vi "sub_Filter_Waveforms_by_Channel_and_Time.vi"(6 "End Time":timestamp, 7 "Start Time":timestamp, 8 "error in":errorcluster, 9 "Channel Key":string, 10 "Waveforms in":T3[](array[typedef]), 11 "daq.io type in":T1={"daq.io ref"=refnum, "daq.io API Base"="http://dashboard.daq.io/api/v1", "Device Key"="", "Account ID"="", "online"=TRUE, "SSL"=TRUE}) -> (0 "error out":errorcluster, 2 "Filtered Waveforms out":T3[](array[typedef]), 3 "daq.io type out":T1={"daq.io ref"=refnum, "daq.io API Base"="http://dashboard.daq.io/api/v1", "Device Key"="", "Account ID"="", "online"=TRUE, "SSL"=TRUE})   [LabVIEW 2013, in "daqio minimal.lvlib"]
doc: "This VI filters existing waveforms by date and channel name and returns only the ones specified by the user. If no start time is specified, all entries before end time will be returned. If no end time is specified, all entries after start time are specified. If neither start nor end time are specified, all entries will be returned. Pass \"*\" as Channel Key if you would like to return all Channels"
uses:
  daqio minimal.lvlib
  _typedefs/daqio-read-waveform-JSON-header-time.ctl
  _typedefs/daqio-Type.ctl
  <vilib>/httpClient/ClientHandle.ctl
  _typedefs/daqio-Device.ctl
  _typedefs/daqio-Channels.ctl
  _typedefs/daqio-Device-Dashboards.ctl
  <vilib>/Easy HTTP Client/Easy HTTP.lvlib
  <vilib>/httpClient/LabVIEWHTTPClient.lvlib
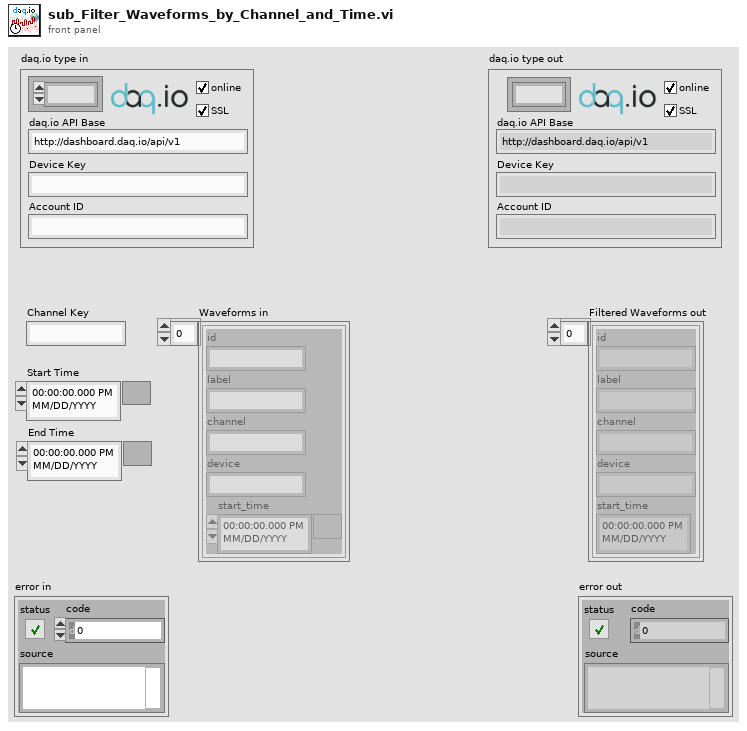
[diagram p1: front panel]
types:
  T1 = typedef "daqio minimal.lvlib/daqio-Type.ctl" = cluster{"daq.io ref":T2, "daq.io API Base":string, "Device Key":string, "Account ID":string, "online":bool, "SSL":bool}
  T2 = typedef "LabVIEWHTTPClient.lvlib/ClientHandle.ctl" = refnum<k1>
  T3 = typedef "daqio minimal.lvlib/daqio-read-waveform-JSON-header-time.ctl" = cluster{"id":string, "label":string, "channel":string, "device":string, "start_time":timestamp}
  T4 = typedef "daqio minimal.lvlib/daqio-Device.ctl" = cluster{"id":string, "label":string, "key":string, "channels":T5[], "tags":cluster{"key":string, "value":string}[], "events":cluster{"id":string, "key":string, "label":string}[], "files":string[], "permissions":cluster{"write":string[], "read":string[]}, "dashboards":T6[]}
  T5 = typedef "daqio minimal.lvlib/daqio-Channels.ctl" = cluster{"key":string, "label":string, "data_type":string, "id":string}
  T6 = typedef "daqio minimal.lvlib/daqio-Device-Dashboards.ctl" = cluster{"active":bool, "definition":string, "_id":string, "label":string}
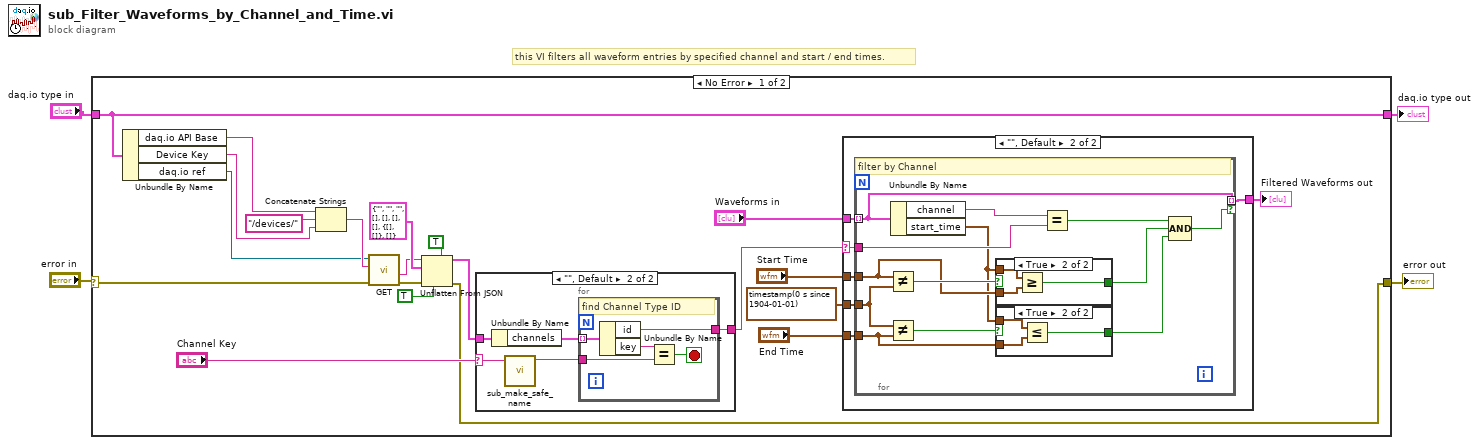
[diagram p0: block diagram]
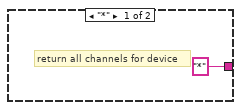
[diagram p2: hidden frame]
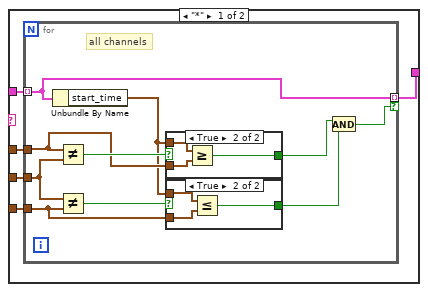
[diagram p3: hidden frame]
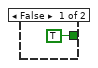
[diagram p4: hidden frame]
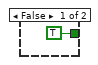
[diagram p5: hidden frame]
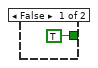
[diagram p6: hidden frame]
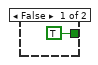
[diagram p7: hidden frame]
diagram:
  # "this VI filters all waveform entries by specified channel and start / end times."
  n1 = case shown="No Error" "error in" {
    selector: "error in" -> [w11 w88]
    tunnel: [w5 w88] -> w3
    tunnel: "daq.io type in" -> [w18 w87]
    tunnel: [w18 w87] -> w1
    frame No Error {
      n2 = Unbundle By Name(w18) -> ("daq.io API Base"=w8:string, "Device Key"=w6:string, "daq.io ref"=w10:T2)
      n3 = Concatenate Strings(w8, "/devices/" ("string"), w6) -> (w17:string)
      n4 = call <vilib>:"GET.vi"("error in (no error)"=w11, "url"=w17, "client handle"=w10) -> ("error out"=w13:errorcluster, "body"=w12:string)  [unwired: 4 in, 3 out]
      n5 = Unflatten From JSON(enable LabVIEW extensions? (T)=TRUE, JSON string=w12, type and defaults=T4 {"id"="", "label"="", "key"="", "channels"=[], "tags"=[], "events"=[], "files"=[], "permissions"={"write"=[], "read"=[]}, "dashboards"=[]} ("Device"), default null elements? (F)=TRUE, error in (no error)=w13) -> (value=w9:T4, error out=w5:errorcluster)  [unwired: 2 in]
      n6 = case shown="\"\", Default" "Channel Key" {
        selector: "Channel Key" -> [_ w30]
        tunnel: ["*" ("id") w28] -> w23
        tunnel: w9 -> [_ w29]
        frame "*" {
          # "return all channels for device"
        }
        frame "", Default {
          n7 = Unbundle By Name(w29) -> ("channels"=w27:T5[])
          n8 = call "sub_make_safe_name.vi"("Input String"=w30) -> ("Safe Output String"=w31:string)  [unwired: 10 in]
          n9 = for {
            tunnel: w31 -> [w36]
            tunnel: [w34] -> w28
            tunnel: w27 -> [w33] mode=indexing
            stop <- w35 stop-if-true
            # "find Channel Type ID"
            n10 = Unbundle By Name(w33) -> ("id"=w34:string, "key"=w32:string)
            n11 = Equal?(x=w32, y=w36) -> (x = y?=w35:bool)
          }
        }
      }
      n12 = case shown="\"\", Default" w23 {
        selector: w23 -> [_ w63]
        tunnel: "Waveforms in" -> [w41 w65]
        tunnel: [w37 w64] -> w24
        tunnel: "Start Time" -> [w40 w62]
        tunnel: "End Time" -> [w39 w61]
        tunnel: timestamp(0 s since 1904-01-01) ("default value 1") -> [w38 w60]
        frame "*" {
          n13 = for {
            tunnel: w41 -> [w45] mode=indexing
            tunnel: w40 -> [w49]
            tunnel: w39 -> [w48]
            tunnel: w38 -> [w47]
            tunnel: [w45] -> w37 mode=indexing if=w42
            # "all channels"
            n14 = Unbundle By Name(w45) -> ("start_time"=w46:timestamp)
            n15 = Not Equal?(x=w49, y=w47) -> (x != y?=w51:bool)
            n16 = Not Equal?(x=w47, y=w48) -> (x != y?=w50:bool)
            n17 = case shown="True" w51 {
              tunnel: w46 -> [_ w59]
              tunnel: w49 -> [_ w58]
              tunnel: [TRUE w57] -> w44
              frame False {
              }
              frame True {
                n18 = Greater Or Equal?(x=w59, y=w58) -> (x >= y?=w57:bool)
              }
            }
            n19 = case shown="True" w50 {
              tunnel: w48 -> [_ w55]
              tunnel: w46 -> [_ w54]
              tunnel: [TRUE w53] -> w43
              frame False {
              }
              frame True {
                n20 = Less Or Equal?(x=w54, y=w55) -> (x <= y?=w53:bool)
              }
            }
            n21 = And(x=w44, y=w43) -> (x .and. y?=w42:bool)
          }
        }
        frame "", Default {
          n22 = for {
            tunnel: w65 -> [w77] mode=indexing
            tunnel: [w77] -> w64 mode=indexing if=w75
            tunnel: w63 -> [w74]
            tunnel: w62 -> [w71]
            tunnel: w61 -> [w70]
            tunnel: w60 -> [w72]
            # "filter by Channel"
            n23 = Not Equal?(x=w71, y=w72) -> (x != y?=w73:bool)
            n24 = Not Equal?(x=w72, y=w70) -> (x != y?=w68:bool)
            n25 = Unbundle By Name(w77) -> ("channel"=w78:string, "start_time"=w69:timestamp)
            n26 = case shown="True" w73 {
              tunnel: w69 -> [_ w86]
              tunnel: w71 -> [_ w85]
              tunnel: [TRUE w84] -> w66
              frame False {
              }
              frame True {
                n27 = Greater Or Equal?(x=w86, y=w85) -> (x >= y?=w84:bool)
              }
            }
            n28 = case shown="True" w68 {
              tunnel: w70 -> [_ w82]
              tunnel: w69 -> [_ w81]
              tunnel: [TRUE w80] -> w67
              frame False {
              }
              frame True {
                n29 = Less Or Equal?(x=w81, y=w82) -> (x <= y?=w80:bool)
              }
            }
            n30 = Equal?(x=w78, y=w74) -> (x = y?=w76:bool)
            n31 = Compound Arithmetic op=AND(w76, w66, w67) -> (w75:bool)
          }
        }
      }
      "Filtered Waveforms out" <- w24
    }
    frame Error {
    }
  }
  "error out" <- w3
  "daq.io type out" <- w1
